vi "DAQ_Init.vi"(0 "Physical Channel X":string="Dev1/ai0", 5 "Physical Channel Y":string="Dev1/ai1", 9 "Samples per Read":i32, 11 "Error in":errorcluster) -> (4 "task":refnum<k21>, 15 "error out":errorcluster)   [LabVIEW 2024]
uses:
  <vilib>/DAQmx/create/channels.llb/DAQmx Create Channel (AI-Voltage-Basic).vi
  <vilib>/DAQmx/configure/timing.llb/DAQmx Timing (Sample Clock).vi
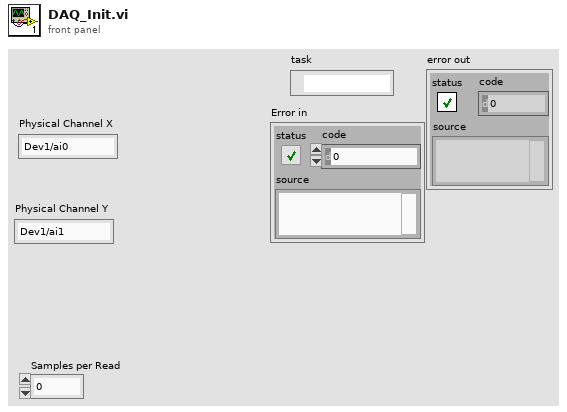
[diagram p1: front panel]
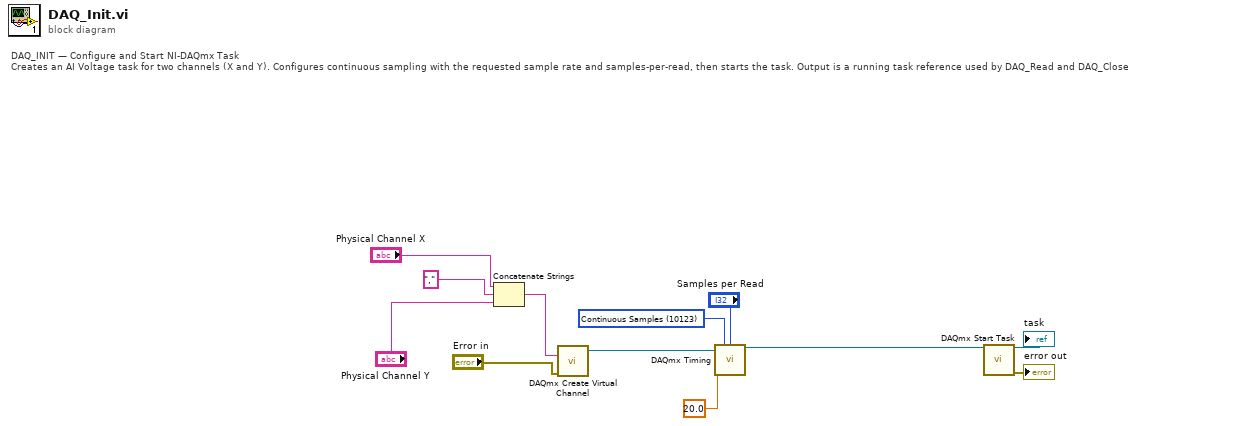
[diagram p0: block diagram]
diagram:
  w2 = 10123 items=["Finite Samples"=10178, "Continuous Samples"=10123, "Hardware Timed Single Point"=12522] ("sample mode")
  # "DAQ_INIT — Configure and Start NI-DAQmx Task\nCreates an AI Voltage task for two channels (X and Y). Configures continuous sampling with the requested sample rate and samples-per-read, then starts the task. Output is a running task reference used by DAQ_Read and DAQ_Close"
  n1 = Concatenate Strings("Physical Channel X", "," ("string"), "Physical Channel Y") -> (w6:string)
  n2 = call-poly <vilib>:"DAQmx Create Virtual Channel.vi"("physical channels"=w6, "error in"="Error in") -> ("task out"=w4:refnum<k21>)  [unwired: 12 in, 1 out]
  n3 = call-poly <vilib>:"DAQmx Timing.vi"("task/channels in"=w4, "sample mode"=w2, "samples per channel"="Samples per Read", "rate"=20.0) -> ("task out"=w12:refnum<k21>)  [unwired: 10 in, 1 out]
  n4 = call <vilib>:"DAQmx Start Task.vi"("task/channels in"=w12) -> ("task out"=→"task":refnum<k21>, "error out"=→"error out":errorcluster)  [unwired: 13 in]
